vi "12Weights-to-4Weights.vi"(0 "output cluster":T1) -> ()   [LabVIEW 2020]
panel:
  in  "Dummy Hidden Weight Bias":dbl[][][][](array[numeric])
  in  "Dummy Hidden Weight Array":dbl[][][][](array[numeric])
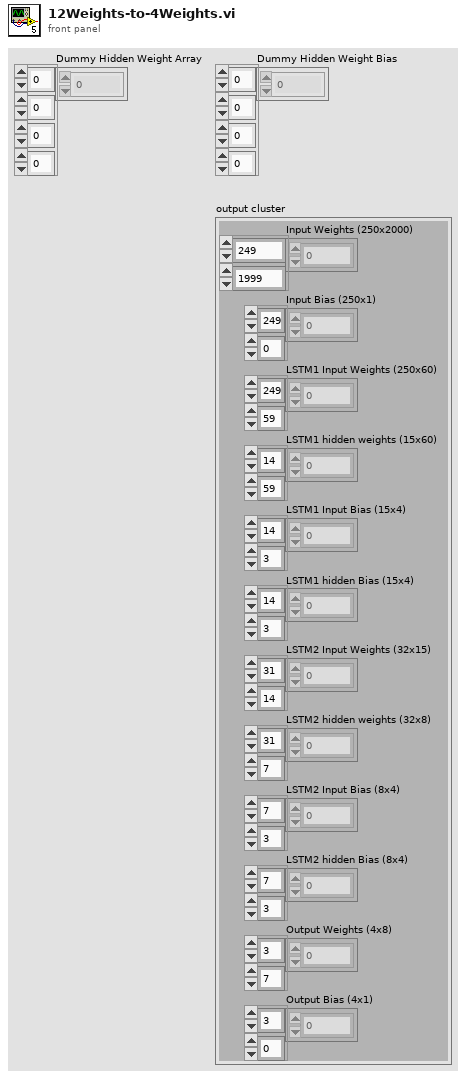
[diagram p1: front panel]
types:
  T1 = cluster{"Input Weights (250x2000)":dbl[][], "Input Bias (250x1)":dbl[][], "LSTM1 Input Weights (250x60)":dbl[][], "LSTM1 hidden weights (15x60)":dbl[][], "LSTM1 Input Bias (15x4)":dbl[][], "LSTM1 hidden Bias (15x4)":dbl[][], "LSTM2 Input Weights (32x15)":dbl[][], "LSTM2 hidden weights (32x8)":dbl[][], "LSTM2 Input Bias (8x4)":dbl[][], "LSTM2 hidden Bias (8x4)":dbl[][], "Output Weights (4x8)":dbl[][], "Output Bias (4x1)":dbl[][]}
  T2 = cluster{"Weights (250x2001)":dbl[][], "Weights (4x4x250x15)":dbl[][][][], "Weights(4x4x15x8)":dbl[][][][], "Weights (4x9)":dbl[][]}
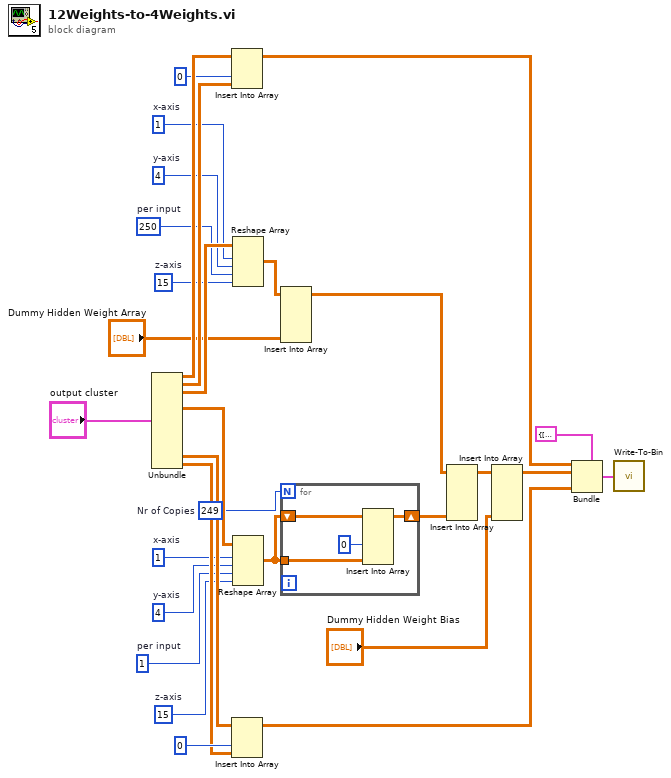
[diagram p0: block diagram]
diagram:
  w13 = 249  # Nr of Copies
  w9 = 1  # per input
  w8 = 15  # z-axis
  w14 = 4  # y-axis
  w15 = 1  # x-axis
  w10 = 250  # per input
  w11 = 15  # z-axis
  w17 = 4  # y-axis
  w18 = 1  # x-axis
  n1 = Unbundle("output cluster") -> ("Input Weights (250x2000)"=w27:dbl[][], "Input Bias (250x1)"=w26:dbl[][], "LSTM1 Input Weights (250x60)"=w19:dbl[][], "LSTM1 Input Bias (15x4)"=w16:dbl[][], "Output Weights (4x8)"=w22:dbl[][], "Output Bias (4x1)"=w21:dbl[][])  [unwired: 6 out]
  n2 = Insert Into Array(array=w27, index (col)=0 ("disabled index (col)"), new element=w26) -> (w24:dbl[][])  [unwired: 1 in]
  n3 = Insert Into Array(array=w22, index (col)=0 ("disabled index (col)"), new element=w21) -> (w20:dbl[][])  [unwired: 1 in]
  n4 = Reshape Array(w19, w18, w17, w10, w11) -> (w7:dbl[][][][])
  n5 = Reshape Array(w16, w15, w14, w9, w8) -> (w12:dbl[][][][])
  n6 = Insert Into Array(array=w7, new element="Dummy Hidden Weight Array") -> (w5:dbl[][][][])  [unwired: 4 in]
  n7 = for {
    N: w13 -> [_]
    shift-right: [w33] -> w4
    shift-left: w12 -> [w34]
    tunnel: w12 -> [w32]
    n8 = Insert Into Array(array=w34, index (dim 2)=0 ("disabled index (col)"), new element=w32) -> (w33:dbl[][][][])  [unwired: 3 in]
  }
  n9 = Insert Into Array(array=w5, new element=w4) -> (w3:dbl[][][][])  [unwired: 4 in]
  n10 = Insert Into Array(array=w3, new element="Dummy Hidden Weight Bias") -> (w1:dbl[][][][])  [unwired: 4 in]
  n11 = Bundle(cluster=T2 {"Weights (250x2001)"=[], "Weights (4x4x250x15)"=[], "Weights(4x4x15x8)"=[], "Weights (4x9)"=[]} ("Weights Cluster"), "Weights (250x2001)"=w24, "Weights (4x4x250x15)"=w1, "Weights (4x9)"=w20) -> (w29:T2)  [unwired: 1 in]
  n12 = call "Write-To-Bin.vi"("Weights Cluster"=w29) -> ()
